vi "Get-KeyValue-Section.vi"(8 "error in (no error)":errorcluster, 9 "Key":string, 10 "Section":string, 11 "Config in":refnum<class "Config.lvclass">) -> (0 "error out":errorcluster, 2 "Value":string, 3 "Config out":refnum<class "Config.lvclass">)   [LabVIEW 2020, in "Config.lvclass"]
uses:
  Config.lvclass
  Config.lvclass/Config.ctl
  <userlib>/_OpenG.lib/dictionary/dictionary.llb/Dictionary Object RefNum__ogtk.ctl
  <userlib>/_OpenG.lib/dictionary/dictionary.llb/Dictionary Object RefNum - Enum__ogtk.ctl
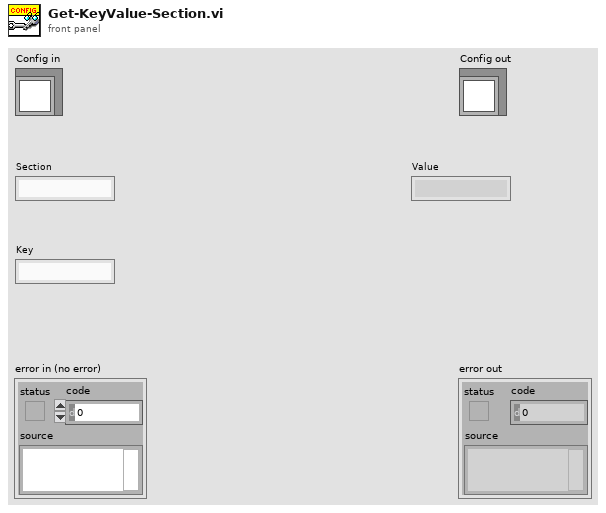
[diagram p1: front panel]
types:
  T1 = typedef "Dictionary Object RefNum__ogtk.ctl" = refnum<k1>
  T2 = cluster{"Keys":string[], "Keys-values":string[]}[]
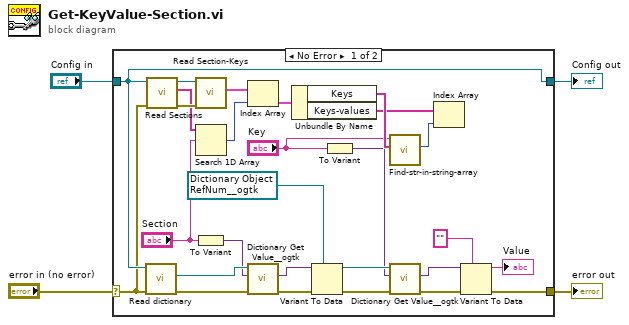
[diagram p0: block diagram]
diagram:
  n1 = case shown="No Error" "error in (no error)" {
    selector: "error in (no error)" -> [w21 w33]
    tunnel: [w8 w33] -> w3
    tunnel: [w22 w32] -> w1
    tunnel: "Config in" -> [w22 w32]
    frame No Error {
      w18 = T1 refnum items=["Dictionary"] ("Object RefNum")
      n2 = call "Read dictionary.vi"("error in (no error)"=w21, "Config in"=w22) -> ("error out"=w20:errorcluster, "Object RefNum"=w19:T1)  [unwired: 7 in, 1 out]
      n3 = call "Read Sections.vi"("error in (no error)"=w21, "Config in"=w22) -> ("error out"=w30:errorcluster, "Sections"=w24:string[], "Config out"=w31:refnum<class "Config.lvclass">)  [unwired: 7 in]
      n4 = call "Read Section-Keys.vi"("error in (no error)"=w30, "Config in"=w31) -> ("Section-Keys"=w29:T2)  [unwired: 7 in, 2 out]
      n5 = Search 1D Array(1D array=w24, element="Section") -> (index of element=w23:i32)  [unwired: 1 in]
      n6 = To Variant(anything="Section") -> (Variant=w15:variant)
      n7 = Index Array(array=w29, index=w23) -> (element=w28:cluster{"Keys":string[], "Keys-values":string[]})
      n8 = call <userlib>:"Dictionary Get Value__ogtk.vi"("error in"=w20, "key"=w15, "dictionary"=w19) -> ("error out"=w16:errorcluster, "value"=w17:variant)  [unwired: 5 in, 2 out]
      n9 = Unbundle By Name(w28) -> ("Keys"=w27:string[], "Keys-values"=w25:string[])
      n10 = Variant To Data(error in=w16, type=w18, Variant=w17) -> (data=w14:T1, error out=w13:errorcluster)
      n11 = To Variant(anything="Key") -> (Variant=w11:variant)
      n12 = call "Find-str-in-string-array.vi"("str array"=w27, "str"="Key") -> ("found index"=w26:i32)  [unwired: 9 in]
      n13 = call <userlib>:"Dictionary Get Value__ogtk.vi"("error in"=w13, "key"=w11, "dictionary"=w14) -> ("error out"=w9:errorcluster, "value"=w10:variant)  [unwired: 5 in, 2 out]
      n14 = Index Array(array=w25, index=w26) -> ()  [unwired: 1 out]
      n15 = Variant To Data(error in=w9, type="" ("Key"), Variant=w10) -> (data=→"Value":string, error out=w8:errorcluster)
    }
    frame Error {
    }
  }
  "error out" <- w3
  "Config out" <- w1
